vi "test-SwerveDrvPoseEst2-ALL-TESTS.vi"(8 "error in (no error)":errorcluster) -> (0 "error out":errorcluster, 3 "All Passed":bool)   [LabVIEW 2019]
panel:
  out "Test 2":bool
  out "Test 1":bool
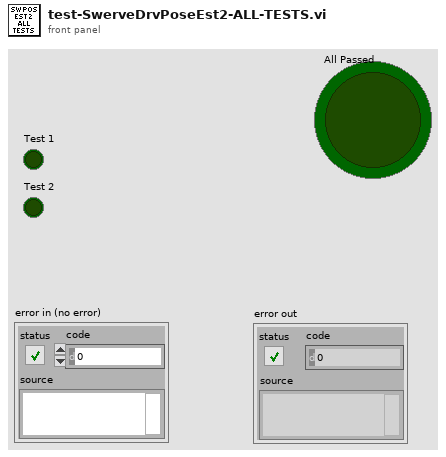
[diagram p1: front panel]
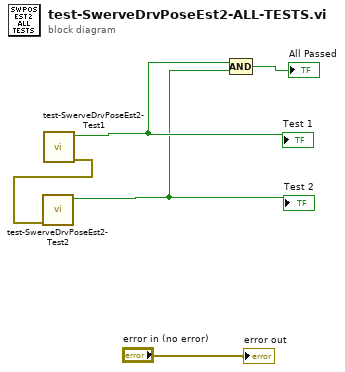
[diagram p0: block diagram]
diagram:
  n1 = call "test-SwerveDrvPoseEst2-Test1.vi"() -> ("error out"=w1:errorcluster, "Test Passed"=w3:bool)  [unwired: 10 in]
  "Test 1" <- w3
  n2 = call "test-SwerveDrvPoseEst2-Test2.vi"("error in (no error)"=w1) -> ("Test Passed"=w2:bool)  [unwired: 9 in, 1 out]
  "Test 2" <- w2
  n3 = Compound Arithmetic op=AND(w3, w2) -> (→"All Passed":bool)
  "error out" <- "error in (no error)"
